vi "Write Name.vi"(7 "Linked List ID":string, 8 "error in (no error)":errorcluster, 10 "Name":string, 11 "Linked List Ref":refnum<data-value>) -> (0 "error out":errorcluster, 3 "Linked List Ref out":refnum<data-value>)   [LabVIEW 2020, in "Linked Lists.lvlib" / "Linked List Ref.lvclass"]
uses:
  <vilib>/gpm_packages/@cs/linked-list/Source/Linked List/Linked List Ref/Linked List Ref.lvclass
  <vilib>/gpm_packages/@cs/linked-list/Source/Linked List/ILinkedList/ILinked List.lvclass
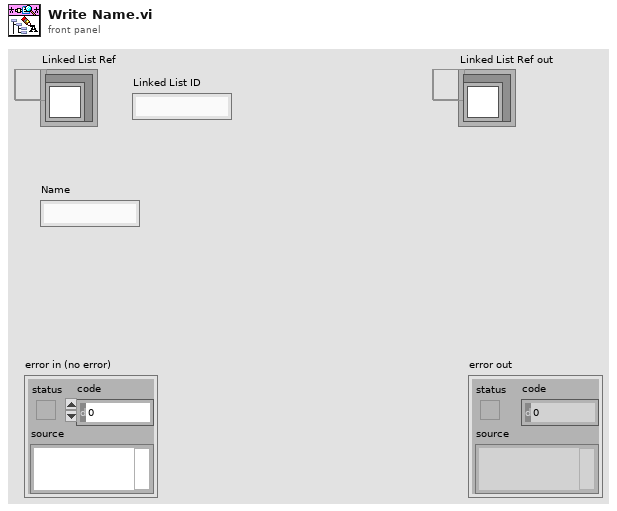
[diagram p1: front panel]
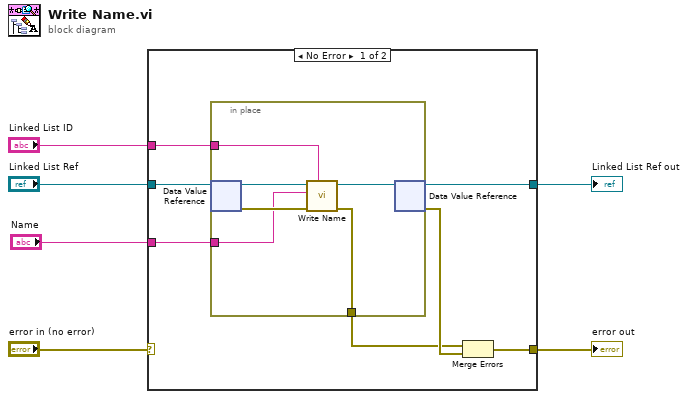
[diagram p0: block diagram]
diagram:
  n1 = case shown="No Error" "error in (no error)" {
    selector: "error in (no error)" -> [_ w21]
    tunnel: "Linked List Ref" -> [w13 w20]
    tunnel: "Linked List ID" -> [w12 _]
    tunnel: [w10 w21] -> w3
    tunnel: [w11 w20] -> w2
    tunnel: "Name" -> [w7 _]
    frame No Error {
      n2 = in-place {
        in-place-border: w12 -> [w15]
        in-place-border: [w16] -> w8
        in-place-border: w7 -> [w14]
        n3 = in-place-dvr #1(w13) -> (w19:refnum<class "ILinked List.lvclass">, w17:errorcluster)
        n4 = call-dynamic "Write Name.vi"("Linked List ID"=w15, "error in (no error)"=w17, "Name"=w14, "ILinked List in"=w19) -> ("error out"=w16:errorcluster, "ILinked List out"=w18:refnum<class "ILinked List.lvclass">)  [unwired: 6 in]
        n5 = in-place-dvr #1(w18) -> (w11:refnum<data-value>, w9:errorcluster)
      }
      n6 = Merge Errors(w8, w9) -> (w10:errorcluster)
    }
    frame Error {
    }
  }
  "error out" <- w3
  "Linked List Ref out" <- w2
